vi "lowPassFilter_v6.vi"(7 "Initialize?":bool, 8 "Sampling Time [s]":fxp<+,25,0>=0.9999999701976776, 9 "2*zeta":fxp<+,16,1>=1.399993896484375, 10 "omega_0 [rad/s]":fxp<+,16,16>, 11 "Input":fxp<+/-,31,7>) -> (0 "Sampling\nTime Out":fxp<+,25,0> format="%.32g", 3 "Output":fxp<+/-,31,7>)   [LabVIEW 2017, in "FPGA Controllers.lvlib"]
doc: "Implements a second-order low-pass filter with damping and natural frequency.\n\nv2: Simplified with Backward Euler for FPGA, implement SCTL\n\nv6: Improved FXP balancing to reduce output width."
uses:
  FPGA Controllers.lvlib
  <vilib>/rvi/FXPMathLib/FxpSub/XNode/nifxpmath_Sub.xnode
  <vilib>/rvi/FXPMathLib/FxpMul/XNode/nifxpmath_Multiplier.xnode
  <vilib>/rvi/FXPMathLib/sim/FxpSim.dll
  <vilib>/rvi/FXPMathLib/FxpAdd/XNode/nifxpmath_Add.xnode
  <vilib>/rvi/FXPMathLib/FxpDiv/XNode/nifxpmath_Div.xnode
  <vilib>/Platform/TimedLoop/XDataNode/XDataNode.xnode
  <vilib>/Platform/TimedLoop/XDataNode/nitl_modes.ctl
  <vilib>/Platform/TimedLoop/XDataNode/XDNodeRunTimeDep.lvlib
  <vilib>/Platform/TimedLoop/XDataNode/wakeup.ctl
  <vilib>/Platform/TimedLoop/XDataNode/timing_clust.ctl
  <vilib>/rvi/FXPMathLib/FxpDiv/simVIs/DllFxpDivTemp_sub.vi
  <vilib>/rvi/FXPMathLib/FxpDiv/subVIs/nifxpmath_Div_SimConfig.ctl
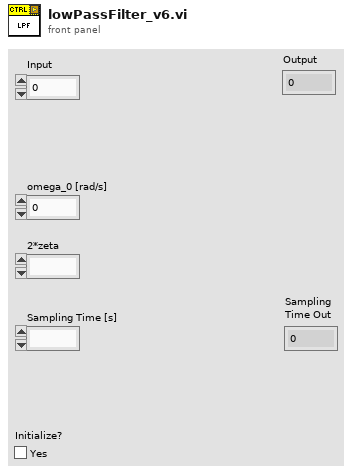
[diagram p1: front panel]
types:
  T1 = typedef "XDNodeRunTimeDep.lvlib/timing_clust.ctl" = cluster{"Expected End [f-1]":u64, "Actual End [f-1]":u64, "Finished Late? [f-1]":bool, "Expected End [i-1]":u64, "Actual End [i-1]":u64, "Finished Late? [i-1]":bool, "Expected Start [i]":u64, "Actual Start [i]":u64, "Expected Start [f]":u64, "Actual Start [f]":u64, "Source Name":string, "Structure Name":string, "Period":i64, "Deadline":i64, "Offset":i64, "Start":i64, "Priority":i32, "Timeout":i32, "Mode":T2, "Wakeup Reason":T3, "Error":errorcluster, "Source Type":string, "Secondary Source Type":string, "Global End Time":u64, "Global Start Time":u64, "Frame Duration":u64, "Iteration Duration":u64, "Assigned CPU":i32, "I/O Scan Engine Mode":u32}
  T2 = typedef "XDNodeRunTimeDep.lvlib/nitl_modes.ctl" = enum32{"No Change", "Process missed periods, maintain original phase", "Discard missed periods, maintain original phase", "Process missed periods, ignore original phase", "Discard missed periods, ignore original phase"}
  T3 = typedef "XDNodeRunTimeDep.lvlib/wakeup.ctl" = enum32{"Normal", "Aborted", "Asynchronous wakeup", "Timing source error", "Timed loop error", "Timeout"}
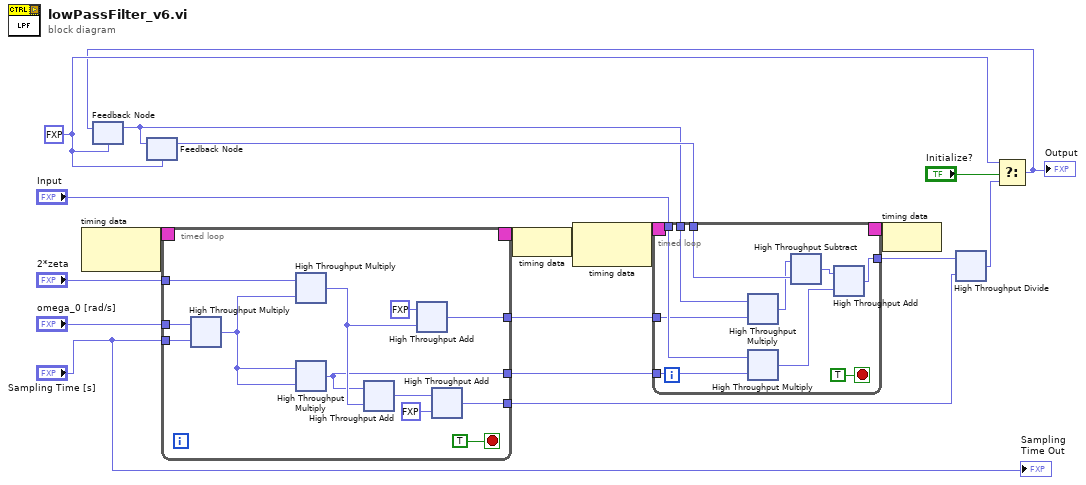
[diagram p0: block diagram]
diagram:
  w15 = fxp<+/-,31,7> 0.0 ("type")
  n1 = node-c288() -> (w4:T1)  [unwired: 1 in]
  n2 = feedback #1(w15) -> (w11:fxp<+/-,31,7>)
  n3 = feedback #2(w15) -> (w12:fxp<+/-,31,7>)
  n4 = feedback-in #2(w11) -> ()
  n5 = timed-loop {
    timing: w4 -> [_]
    timing-out: [_] -> w3
    tunnel: "omega_0 [rad/s]" -> [w30]
    tunnel: "2*zeta" -> [w29]
    tunnel: "Sampling Time [s]" -> [w28]
    tunnel: [w26] -> w9
    tunnel: [w21] -> w8
    tunnel: [w20] -> w6
    stop <- TRUE stop-if-true
    n6 = xnode ("High Throughput Multiply")("x"=w30, "y"=w28) -> ("x*y"=w23:fxp<+,24,0>)
    n7 = xnode ("High Throughput Multiply")("x"=w29, "y"=w23) -> ("x*y"=w22:fxp<+,25,1>)
    n8 = xnode ("High Throughput Multiply")("x"=w23, "y"=w23) -> ("x*y"=w21:fxp<+,25,0>)
    n9 = xnode ("High Throughput Add")("x"=w21, "y"=w22) -> ("x+y"=w25:fxp<+,27,2>)
    n10 = xnode ("High Throughput Add")("x"=fxp<+,1,2> 2.0, "y"=w22) -> ("x+y"=w26:fxp<+,27,3>)
    n11 = xnode ("High Throughput Add")("x"=w25, "y"=fxp<+,1,1> 1.0) -> ("x+y"=w20:fxp<+,28,3>)
  }
  n12 = node-c288(w3) -> ()
  n13 = node-c288() -> (w2:T1)  [unwired: 1 in]
  n14 = timed-loop {
    timing: w2 -> [_]
    timing-out: [_] -> w1
    tunnel: "Input" -> [w42]
    tunnel: w12 -> [w41]
    tunnel: w11 -> [w40]
    tunnel: w9 -> [w38]
    tunnel: w8 -> [w37]
    tunnel: [w34] -> w7
    stop <- TRUE stop-if-true
    n15 = xnode ("High Throughput Multiply")("x"=w40, "y"=w38) -> ("x*y"=w35:fxp<+/-,35,10>)
    n16 = xnode ("High Throughput Multiply")("x"=w42, "y"=w37) -> ("x*y"=w36:fxp<+/-,31,7>)
    n17 = xnode ("High Throughput Subtract")("x"=w35, "y"=w41) -> ("x-y"=w39:fxp<+/-,36,11>)
    n18 = xnode ("High Throughput Add")("x"=w39, "y"=w36) -> ("x+y"=w34:fxp<+/-,37,12>)
  }
  n19 = node-c288(w1) -> ()
  n20 = xnode "High Throughput Divide"("x"=w7, "y"=w6) -> ("x/y"=w5:fxp<+/-,31,7>)
  n21 = Select(t=w15, s="Initialize?", f=w5) -> (s? t:f=w13:fxp<+/-,31,7>)
  "Output" <- w13
  n22 = feedback-in #1(w13) -> ()
  "Sampling\nTime Out" <- "Sampling Time [s]"
